vi "UI.Menu.Config.State.Set.vi"(8 "error in (no error)":errorcluster, 10 "Enabled":bool, 11 "menu reference":refnum<k9>) -> (0 "error out":errorcluster)   [LabVIEW 2019, in "Instrument Workspace Shared.lvlib"]
uses:
  Instrument Workspace Shared.lvlib
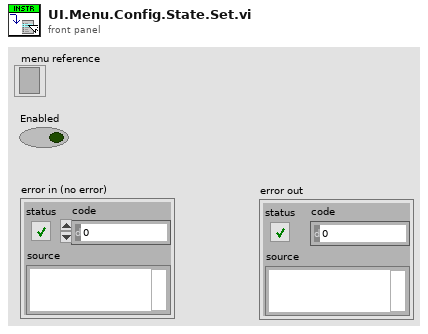
[diagram p1: front panel]
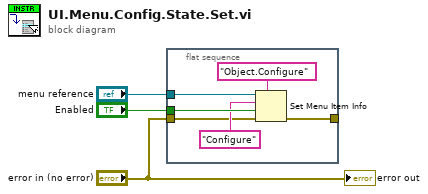
[diagram p0: block diagram]
diagram:
  n1 = flat-sequence {
    tunnel: "Enabled" -> [w9]
    tunnel: "menu reference" -> [w6]
    tunnel: "error in (no error)" -> [w5]
    tunnel: [w4] -> _
    frame #0 {
      n2 = Set Menu Item Info(7:"Object.Configure" ("item tag"), 8:w5, 9:w9, 10:"Configure" ("item name"), 11:w6) -> (0:w4:errorcluster)  [unwired: 2 in, 1 out]
    }
  }
  "error out" <- "error in (no error)"
